vi "Process Data.vi"(8 "error in (no error)":errorcluster, 10 "Raw Pulse In":dbl[](array[numeric]), 11 "DigitiserActor in":refnum<class "DigitiserActor.lvclass">) -> (0 "error out":errorcluster, 3 "DigitiserActor out":refnum<class "DigitiserActor.lvclass">)   [LabVIEW 2019, in "DigitiserActor.lvlib" / "DigitiserActor.lvclass"]
uses:
  DigitiserActor.lvclass
  DigitiserActor.lvclass/DigitiserActor.ctl
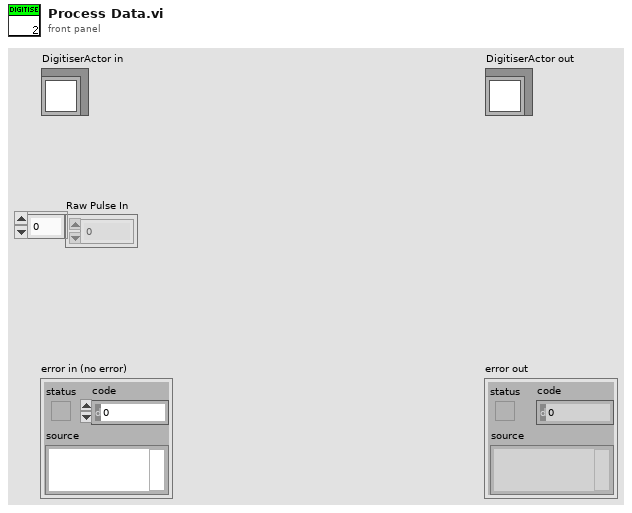
[diagram p1: front panel]
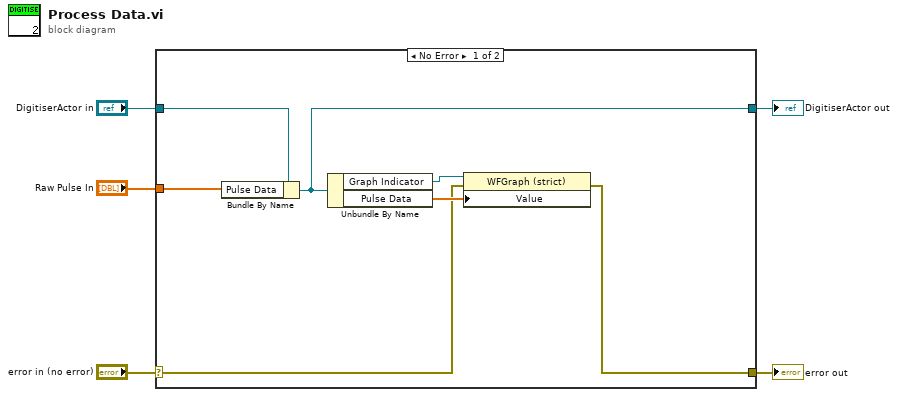
[diagram p0: block diagram]
diagram:
  n1 = case shown="No Error" "error in (no error)" {
    selector: "error in (no error)" -> [w7 w14]
    tunnel: [w6 w14] -> w4
    tunnel: [w10 w13] -> w2
    tunnel: "DigitiserActor in" -> [w11 w13]
    tunnel: "Raw Pulse In" -> [w12 _]
    frame No Error {
      n2 = Bundle By Name(cluster=w11, "Pulse Data"=w12) -> (w10:refnum<class "DigitiserActor.lvclass">)
      n3 = Unbundle By Name(w10) -> ("Graph Indicator"=w9:refnum<vi>, "Pulse Data"=w8:dbl[])
      n4 = property class="WFGraph (strict)"(reference=w9, error in=w7, "Value"=w8) -> (error out=w6:errorcluster)  [unwired: 1 out]
    }
    frame Error {
    }
  }
  "error out" <- w4
  "DigitiserActor out" <- w2
